vi "Update FIFO Full Flag - 32-bit Address.vi"(0 "full in":bool, 5 "full count in":u32, 7 "write":bool, 9 "read":bool, 11 "fifo depth":T1=10 items=["4"=2, "8"=3, "16"=4, "32"=5, "64"=6, "128"=7, "256"=8, "512"=9, "1024"=10, "2048"=11, "4096"=12, "8192"=13, "16384"=14, "32768"=15, "65536"=16, "131072"=17, "262144"=18, "524288"=19, "1048576"=20, "2097152"=21, "4194304"=22, "8388608"=23, "16777216"=24, "33554432"=25, "67108864"=26, "134217728"=27, "268435456"=28, "536870912"=29, "1073741824"=30, "2147483648"=31, "4294967296"=32]) -> (4 "full out":bool, 6 "full count out":u32)   [LabVIEW 2012, in "FIFO.lvlib"]
uses:
  <userlib>/FPGA Library/Code Development/DRAM/RF-RIO/FIFO/FIFO/FPGA/FIFO.lvlib
  <userlib>/FPGA Library/Code Development/DRAM/RF-RIO/FIFO/FIFO/FPGA/Private/FIFO Depth - 32-bit Address.ctl
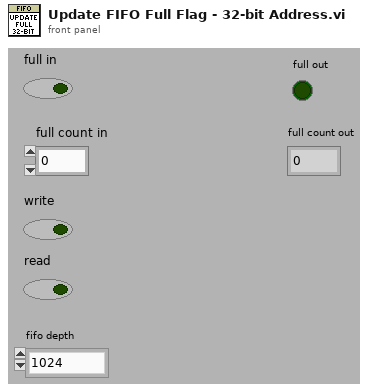
[diagram p1: front panel]
types:
  T1 = typedef "FIFO.lvlib/FIFO Depth - 32-bit Address.ctl" = u8
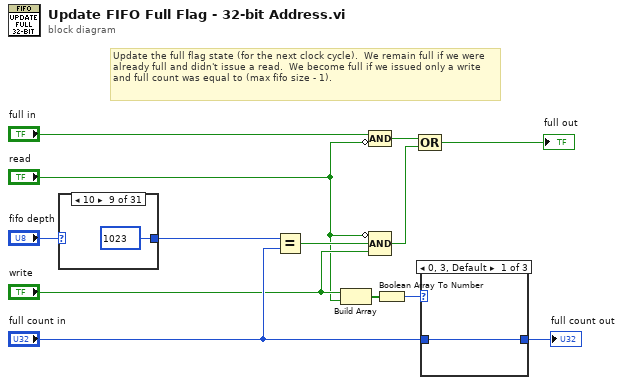
[diagram p0: block diagram]
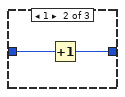
[diagram p2: hidden frame]
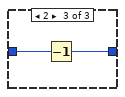
[diagram p3: hidden frame]
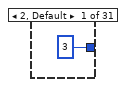
[diagram p4: hidden frame]
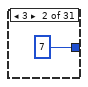
[diagram p5: hidden frame]
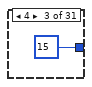
[diagram p6: hidden frame]
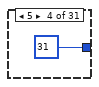
[diagram p7: hidden frame]
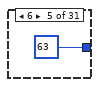
[diagram p8: hidden frame]
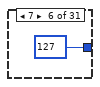
[diagram p9: hidden frame]
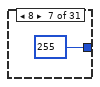
[diagram p10: hidden frame]
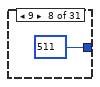
[diagram p11: hidden frame]
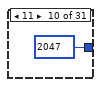
[diagram p12: hidden frame]
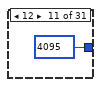
[diagram p13: hidden frame]
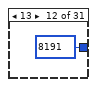
[diagram p14: hidden frame]
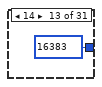
[diagram p15: hidden frame]
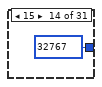
[diagram p16: hidden frame]
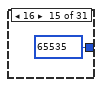
[diagram p17: hidden frame]
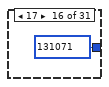
[diagram p18: hidden frame]
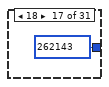
[diagram p19: hidden frame]
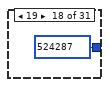
[diagram p20: hidden frame]
diagram:
  # "Update the full flag state (for the next clock cycle).  We remain full if we were already full and didn't issue a read.  We become full if we issued only a write and full count was equal to (max fifo size - 1)."
  n1 = case shown="10" "fifo depth" {
    tunnel: [u32 3 u32 7 u32 15 u32 31 u32 63 u32 127 u32 255 u32 511 u32 1023 u32 2047 u32 4095 u32 8191 u32 16383 u32 32767 u32 65535 u32 131071 u32 262143 u32 524287 u32 1048575 u32 2097151 u32 4194303 u32 8388607 u32 16777215 u32 33554431 u32 67108863 u32 134217727 u32 268435455 u32 536870911 u32 1073741823 u32 2147483647 u32 4294967295] -> w7
    frame 2, Default {
    }
    frame 3 {
    }
    frame 4 {
    }
    frame 5 {
    }
    frame 6 {
    }
    frame 7 {
    }
    frame 8 {
    }
    frame 9 {
    }
    frame 10 {
    }
    frame 11 {
    }
    frame 12 {
    }
    frame 13 {
    }
    frame 14 {
    }
    frame 15 {
    }
    frame 16 {
    }
    frame 17 {
    }
    frame 18 {
    }
    frame 19 {
    }
    frame 20 {
    }
    frame 21 {
    }
    frame 22 {
    }
    frame 23 {
    }
    frame 24 {
    }
    frame 25 {
    }
    frame 26 {
    }
    frame 27 {
    }
    frame 28 {
    }
    frame 29 {
    }
    frame 30 {
    }
    frame 31 {
    }
    frame 32 {
    }
  }
  n2 = Equal?(x=w7, y="full count in") -> (x = y?=w13:bool)
  n3 = Build Array("write", "read") -> (w6:bool[])
  n4 = Compound Arithmetic op=AND("full in", invert "read") -> (w12:bool)
  n5 = Compound Arithmetic op=AND(invert "read", w13, "write") -> (w11:bool)
  n6 = Boolean Array To Number(Boolean array=w6) -> (number=w5:u8)
  n7 = Compound Arithmetic op=OR(w12, w11) -> (→"full out":bool)
  n8 = case shown="0, 3, Default" w5 {
    tunnel: "full count in" -> [w45 w47 w49]
    tunnel: [w45 w46 w48] -> w4
    frame 0, 3, Default {
    }
    frame 1 {
      n9 = Increment(x=w47) -> (x+1=w46:u32)
    }
    frame 2 {
      n10 = Decrement(x=w49) -> (x-1=w48:u32)
    }
  }
  "full count out" <- w4
